vi "GA_Main_Map_ini.vi"(11 "reference":refnum<vi>) -> ()   [LabVIEW 2018]
uses:
  GA_Global.vi
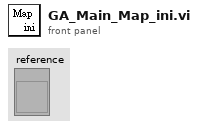
[diagram p1: front panel]
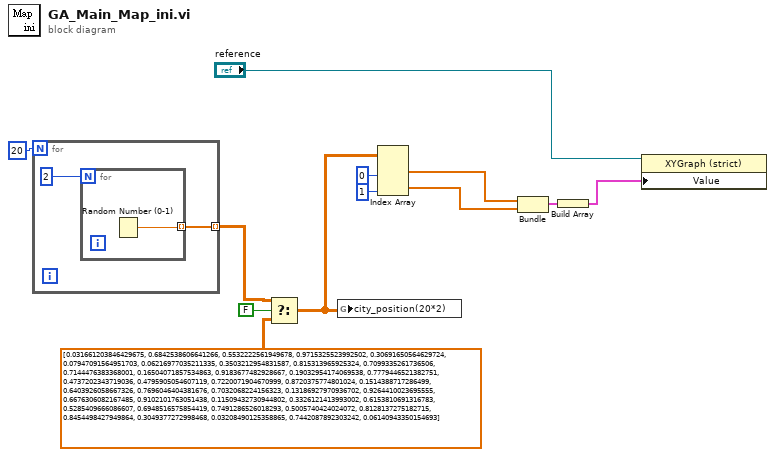
[diagram p0: block diagram]
diagram:
  n1 = for {
    N: 20 -> [_]
    tunnel: [w14] -> w6 mode=indexing
    n2 = for {
      N: 2 -> [_]
      tunnel: [w15] -> w14 mode=indexing
      n3 = Random Number (0-1)() -> (number: 0 to 1=w15:dbl)
    }
  }
  n4 = Select(t=w6, s=FALSE, f=dbl[][] [[0.031661203846429675, 0.6842538606641266], [0.5532222561949678, 0.9715325523992502], [0.30691650564629724, 0.07947091564951703], [0.06216977035211335, 0.3503212954831587], [0.815313965925324, 0.7099335261736506], [0.7144476383368001, 0.16504071857534863], [0.9183677482928667, 0.19032954174069538], [0.7779446521382751, 0.4737202343719036], [0.4795905054607119, 0.7220071904670999], [0.8720375774801024, 0.1514388717286499], [0.6403926058667326, 0.7696046404381676], [0.7032068224156323, 0.13186927970936702], [0.9264410023695555, 0.6676306082167485], [0.9102101763051438, 0.11509432730944802], [0.3326121413993002, 0.6153810691316783], [0.5285409666086607, 0.6948516575854419], [0.7491286526018293, 0.5005740424024072], [0.8128137275182715, 0.8454498427949864], [0.3049377272998468, 0.03208490125358865], [0.7442087892303242, 0.06140943350154693]] ("Array 2")) -> (s? t:f=w1:dbl[][])
  n5 = global write "GA_Global.vi" "city_position(20*2)"(w1) -> ()
  n6 = Index Array "Index Array"(array=w1, index (col) #1=0 ("disabled index (col)"), index (col) #2=1 ("index (col)")) -> (element #1=w11:dbl[], element #2=w8:dbl[])  [unwired: 2 in]
  n7 = Bundle("Array 2"=w11, "Array 2"=w8) -> (w7:cluster{"Array 2":dbl[], "Array 2":dbl[]})  [unwired: 1 in]
  n8 = Build Array(w7) -> (w2:cluster{"Array 2":dbl[], "Array 2":dbl[]}[])
  n9 = property class="XYGraph (strict)"(reference="reference", "Value"=w2) -> ()  [unwired: 1 in, 2 out]
